vi "Initialise camera properties.vi"(8 "error in (no error)":errorcluster, 11 "DAQOrcaFlash in":refnum<class "DAQOrcaFlash.lvclass">) -> (0 "error out":errorcluster, 3 "DAQOrcaFlash out":refnum<class "DAQOrcaFlash.lvclass">)   [LabVIEW 2012, in "DAQOrcaFlash.lvclass"]
uses:
  DAQOrcaFlash.lvclass
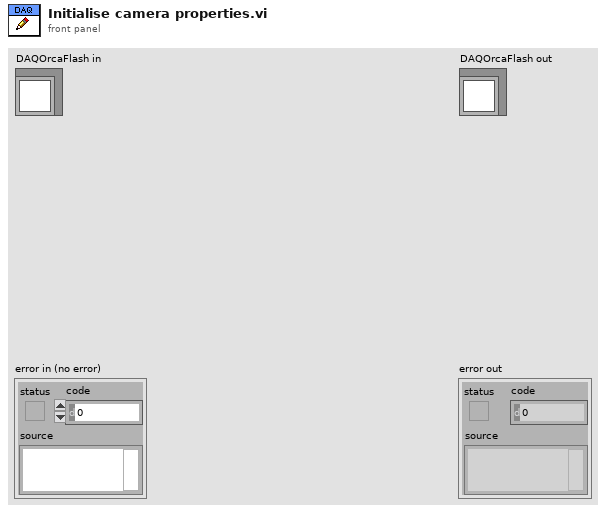
[diagram p1: front panel]
types:
  T1 = typedef "DAQOrcaFlash.lvclass/sensor_mode.ctl" = sgl
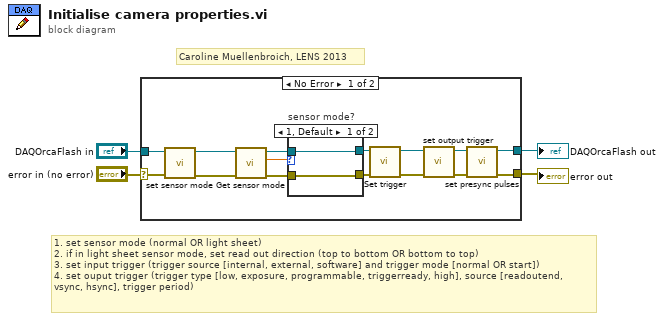
[diagram p0: block diagram]
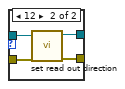
[diagram p2: hidden frame]
diagram:
  # "Caroline Muellenbroich, LENS 2013"
  # "1. set sensor mode (normal OR light sheet)\n2. if in light sheet sensor mode, set read out direction (top to bottom OR bottom to top)\n3. set input trigger (trigger source [internal, external, software] and trigger mode [normal OR start]) \n4. set ouput trigger (trigger type [low, exposure, programmable, triggerready, high], source [readoutend, vsync, hsync], trigger period)"
  n1 = case shown="No Error" "error in (no error)" {
    selector: "error in (no error)" -> [w19 w27]
    tunnel: [w5 w27] -> w1
    tunnel: [w7 w26] -> w2
    tunnel: "DAQOrcaFlash in" -> [w18 w26]
    frame No Error {
      n2 = call-dynamic "set sensor mode.vi"("error in (no error)"=w19, "DAQOrcaFlash in"=w18) -> ("error out"=w13:errorcluster, "DAQOrcaFlash out"=w11:refnum<class "DAQOrcaFlash.lvclass">)  [unwired: 8 in]
      n3 = call-dynamic "Get sensor mode.vi"("error in (no error)"=w13, "DAQOrcaFlash in"=w11) -> ("error out"=w12:errorcluster, "Sensor mode"=w9:T1, "DAQOrcaFlash out"=w10:refnum<class "DAQOrcaFlash.lvclass">)  [unwired: 7 in]
      n4 = case "sensor mode?" shown="1, Default" w9 {
        tunnel: w12 -> [w21 w25]
        tunnel: w10 -> [w20 w24]
        tunnel: [w20 w23] -> w15
        tunnel: [w21 w22] -> w14
        frame 1, Default {
        }
        frame 12 {
          n5 = call-dynamic "set read out direction.vi"("error in (no error)"=w25, "DAQOrcaFlash in"=w24) -> ("error out"=w22:errorcluster, "DAQOrcaFlash out"=w23:refnum<class "DAQOrcaFlash.lvclass">)  [unwired: 8 in]
        }
      }
      n6 = call-dynamic "Set trigger.vi"("error in (no error)"=w14, "DAQOrcaFlash in"=w15) -> ("error out"=w16:errorcluster, "DAQOrcaFlash out"=w17:refnum<class "DAQOrcaFlash.lvclass">)  [unwired: 8 in]
      n7 = call-dynamic "set output trigger.vi"("error in (no error)"=w16, "DAQOrcaFlash in"=w17) -> ("error out"=w6:errorcluster, "DAQOrcaFlash out"=w8:refnum<class "DAQOrcaFlash.lvclass">)  [unwired: 8 in]
      n8 = call-dynamic "set presync pulses.vi"("error in (no error)"=w6, "DAQOrcaFlash in"=w8) -> ("error out"=w5:errorcluster, "DAQOrcaFlash out"=w7:refnum<class "DAQOrcaFlash.lvclass">)  [unwired: 8 in]
    }
    frame Error {
    }
  }
  "error out" <- w1
  "DAQOrcaFlash out" <- w2
